vi "LEDcolorFromDashboard.vi"() -> (2 "LED color":T1)   [LabVIEW 2016]
uses:
  <vilib>/Rock Robotics/Network Tables/NT Read Number.vi
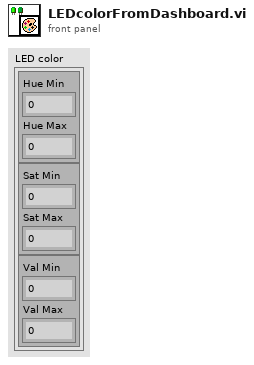
[diagram p1: front panel]
types:
  T1 = cluster{cluster{"Hue Min":dbl, "Hue Max":dbl}, cluster{"Sat Min":dbl, "Sat Max":dbl}, cluster{"Val Min":dbl, "Val Max":dbl}}
  T2 = cluster{cluster{"Numeric":dbl, "Numeric":dbl}, cluster{"Numeric":dbl, "Numeric":dbl}, cluster{"Numeric":dbl, "Numeric":dbl}}
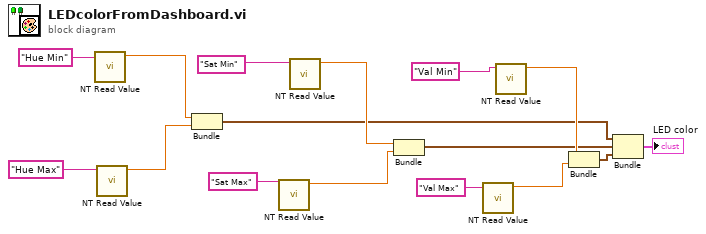
[diagram p0: block diagram]
diagram:
  n1 = call-poly <vilib>:"NT Read Value.vi"("Name"="Hue Min" ("section")) -> ("Numeric"=w10:dbl)  [unwired: 9 in, 1 out]
  n2 = call-poly <vilib>:"NT Read Value.vi"("Name"="Hue Max" ("section")) -> ("Numeric"=w9:dbl)  [unwired: 9 in, 1 out]
  n3 = Bundle("Numeric"=w10, "Numeric"=w9) -> (w2:cluster{"Numeric":dbl, "Numeric":dbl})  [unwired: 1 in]
  n4 = call-poly <vilib>:"NT Read Value.vi"("Name"="Sat Max" ("section")) -> ("Numeric"=w7:dbl)  [unwired: 9 in, 1 out]
  n5 = call-poly <vilib>:"NT Read Value.vi"("Name"="Sat Min" ("section")) -> ("Numeric"=w8:dbl)  [unwired: 9 in, 1 out]
  n6 = Bundle("Numeric"=w8, "Numeric"=w7) -> (w3:cluster{"Numeric":dbl, "Numeric":dbl})  [unwired: 1 in]
  n7 = call-poly <vilib>:"NT Read Value.vi"("Name"="Val Max" ("section")) -> ("Numeric"=w5:dbl)  [unwired: 9 in, 1 out]
  n8 = call-poly <vilib>:"NT Read Value.vi"("Name"="Val Min" ("section")) -> ("Numeric"=w6:dbl)  [unwired: 9 in, 1 out]
  n9 = Bundle("Numeric"=w6, "Numeric"=w5) -> (w4:cluster{"Numeric":dbl, "Numeric":dbl})  [unwired: 1 in]
  n10 = Bundle(w2, w3, w4) -> (→"LED color":T2)  [unwired: 1 in]
